vi "Aero_tunnel_monitor_on_OGI.vi"() -> ()   [LabVIEW 2018]
uses:
  Controls/Post_Process.ctl
  <vilib>/Platform/TimedLoop/XDataNode/timing_clust.ctl
  <vilib>/Platform/TimedLoop/XDataNode/nitl_modes.ctl
  <vilib>/Platform/TimedLoop/XDataNode/wakeup.ctl
  ADAM Client/Sub VIs/ADAM Controls/Update_scan_value.ctl
  Globals/Meas_global.vi
  <vilib>/Utility/file.llb/Write Delimited Spreadsheet (DBL).vi
  <vilib>/Platform/TimedLoop/XDataNode/XDataNode.xnode
  <vilib>/Platform/TimedLoop/XDataNode/XDNodeRunTimeDep.lvlib
panel:
  in  "Filename":path
  in  "Duration in Seconds":dbl=30.0
  in  "Log Full Res Balance data":bool
  in  "Use Polynomial for Ratio":bool
  in  "Manual Ratio":dbl=1.0075
  in  "Display Graph?":bool
  in  "Menu Ring":u16(ring) items=["Lift", "Pitch", "Drag", "Side", "Yaw", "Roll"]
  in  "Samples":i32=1000
  out "Waveform Chart":dbl[](graph)
  in  "Output Roll":bool
  out "Roll":string="0.0 Nm"
  in  "Output Yaw":bool
  out "Yaw":string="0.0 Nm"
  in  "Output Pitch":bool
  out "Pitch":string="0.0 Nm"
  in  "Output SF":bool
  out "SF":string="0.0 N"
  in  "Output Drag":bool
  out "Drag":string="0.0 N"
  in  "Output Lift":bool
  out "Lift":string="0.0 N"
  in  "Balance Safety limits":T1(array[cluster])=[{"Max +ve Range"=80, "Max -ve Range"=80, "Axis"="Lift"}, {"Max +ve Range"=80, "Max -ve Range"=80, "Axis"="Pitch"}, {"Max +ve Range"=80, "Max -ve Range"=80, "Axis"="Drag"}, {"Max +ve Range"=80, "Max -ve Range"=80, "Axis"="Side-Force"}, {"Max +ve Range"=99, "Max -ve Range"=99, "Axis"="Yaw"}, {"Max +ve Range"=80, "Max -ve Range"=80, "Axis"="Roll"}] {"Max -ve Range" min=0 max=125; "Max +ve Range" min=0 max=125}
  out "Monitor Speed (Hz)":dbl
  out "Belt slip warning":bool
  out "Road Status":string="???"
  in  "GotoYaw":bool
  in  "NewYawPos":dbl
  out "YAW POSITION":dbl
  out "Required WindSpeedRatio":dbl
  out "ROAD SPEED m/s":dbl
  in  "BL Fan1":i32
  in  "BL Fan2":i32
  in  "Stop drive":bool
  in  "Start Drive":bool
  in  "Synch to Wind":bool
  out "Road Info":string="???"
  in  "stop":bool
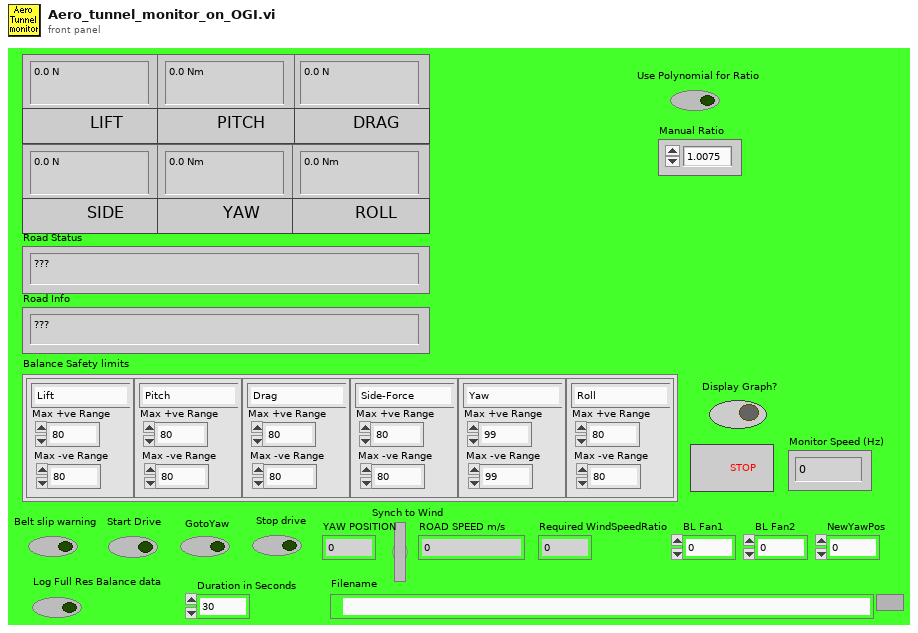
[diagram p1: front panel]
types:
  T1 = cluster{"Max +ve Range":i32, "Max -ve Range":i32, "Axis":string}[]
  T2 = typedef "Post_Process.ctl" = enum16{"Take New Data", "Post Process Raw Data File"}
  T3 = typedef "XDNodeRunTimeDep.lvlib/timing_clust.ctl" = cluster{"Expected End [f-1]":u64, "Actual End [f-1]":u64, "Finished Late? [f-1]":bool, "Expected End [i-1]":u64, "Actual End [i-1]":u64, "Finished Late? [i-1]":bool, "Expected Start [i]":u64, "Actual Start [i]":u64, "Expected Start [f]":u64, "Actual Start [f]":u64, "Source Name":string, "Structure Name":string, "Period":i64, "Deadline":i64, "Offset":i64, "Start":i64, "Priority":i32, "Timeout":i32, "Mode":T4, "Wakeup Reason":T5, "Error":errorcluster, "Source Type":string, "Secondary Source Type":string, "Global End Time":u64, "Global Start Time":u64, "Frame Duration":u64, "Iteration Duration":u64, "Assigned CPU":i32, "I/O Scan Engine Mode":u32}
  T4 = typedef "XDNodeRunTimeDep.lvlib/nitl_modes.ctl" = enum32{"No Change", "Process missed periods, maintain original phase", "Discard missed periods, maintain original phase", "Process missed periods, ignore original phase", "Discard missed periods, ignore original phase"}
  T5 = typedef "XDNodeRunTimeDep.lvlib/wakeup.ctl" = enum32{"Normal", "Aborted", "Asynchronous wakeup", "Timing source error", "Timed loop error", "Timeout"}
  T6 = typedef "Update_scan_value.ctl" = cluster{"Channel Name":string, "New Value":dbl}
  T7 = cluster{"Max +ve Range":i32, "Max -ve Range":i32, "Axis":string}
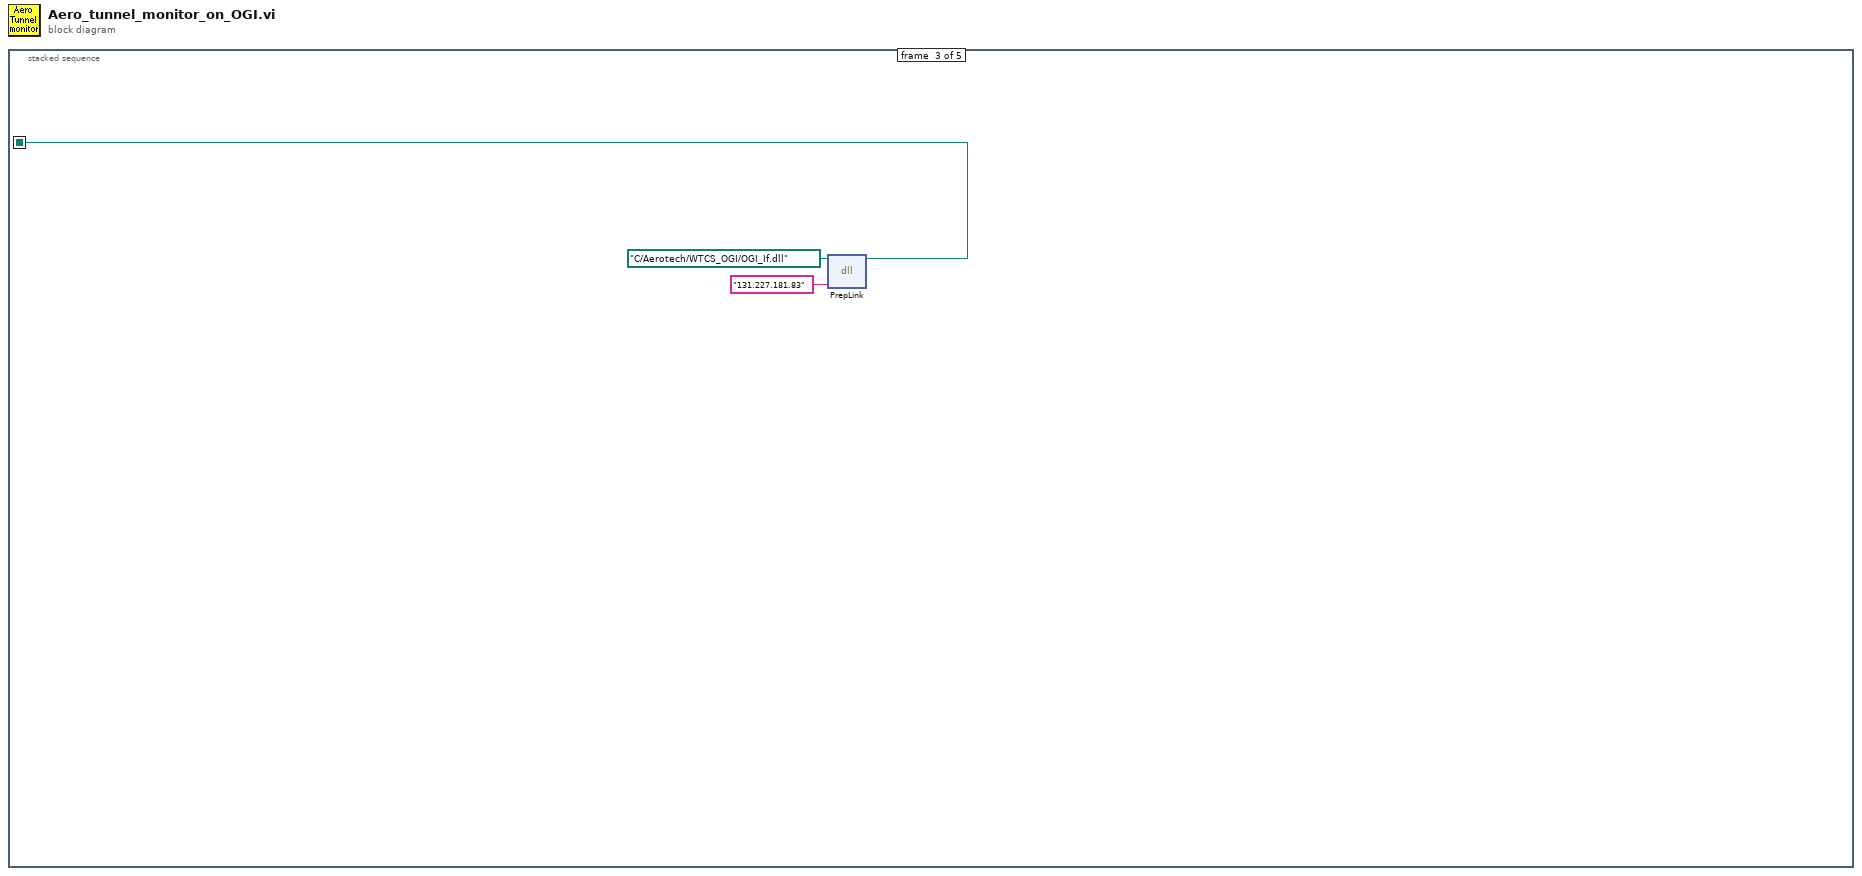
[diagram p0: block diagram]
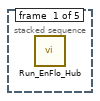
[diagram p2: hidden frame]
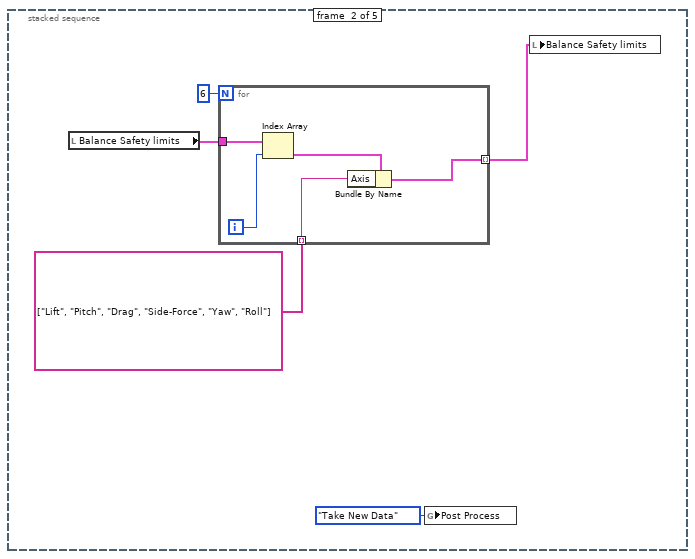
[diagram p3: hidden frame]
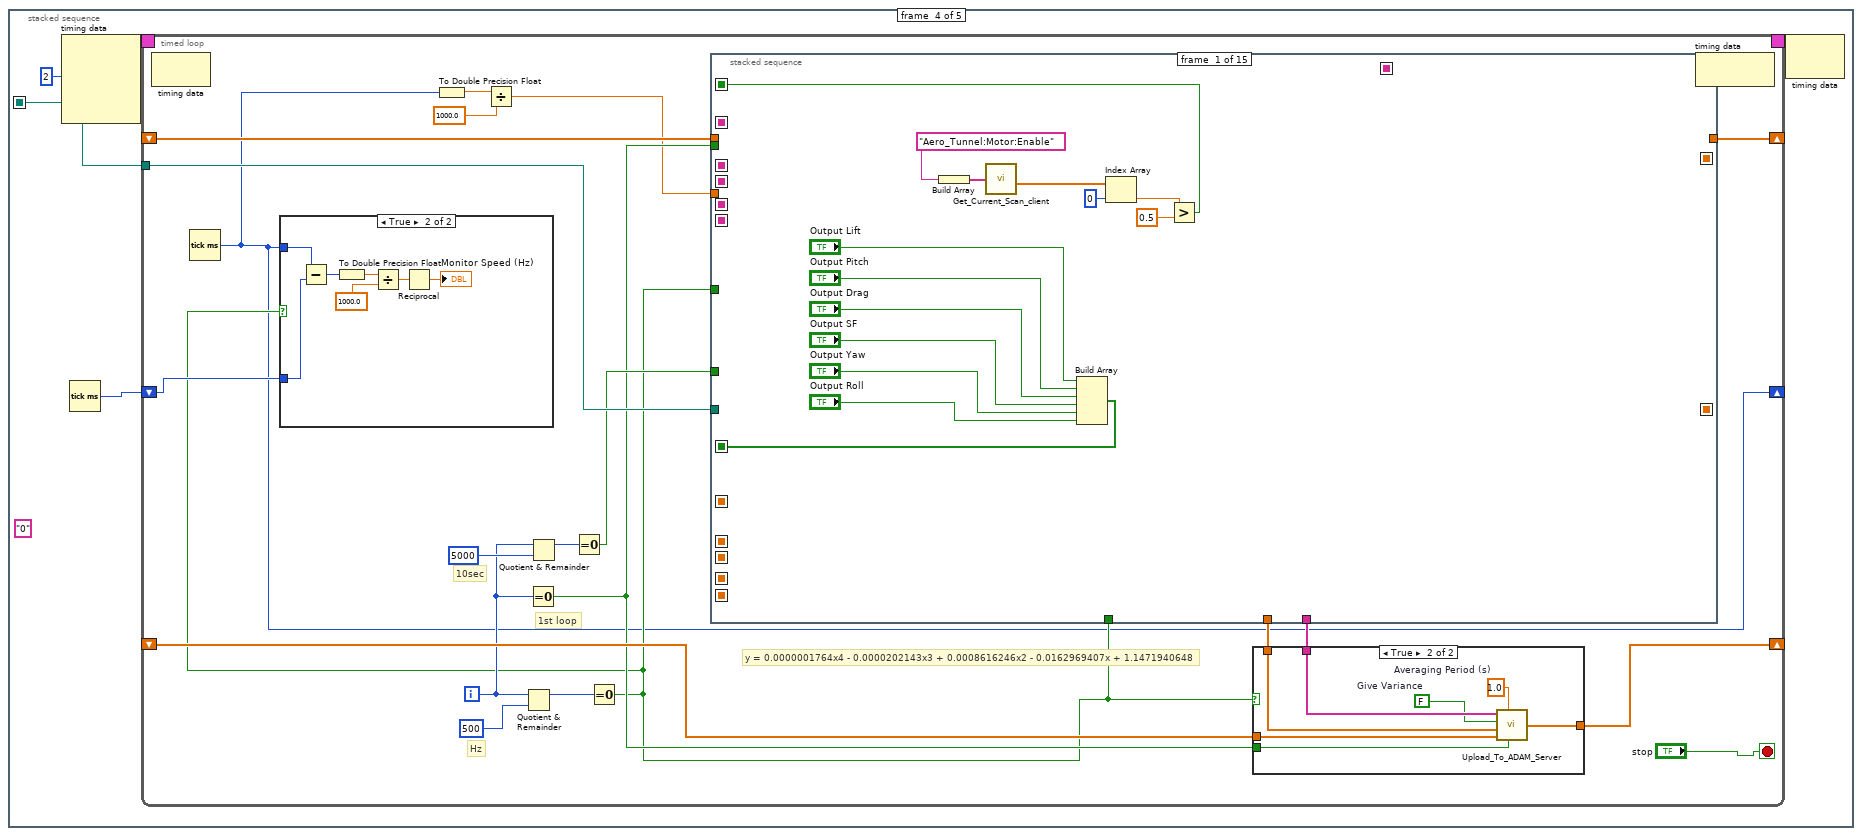
[diagram p4: hidden frame]
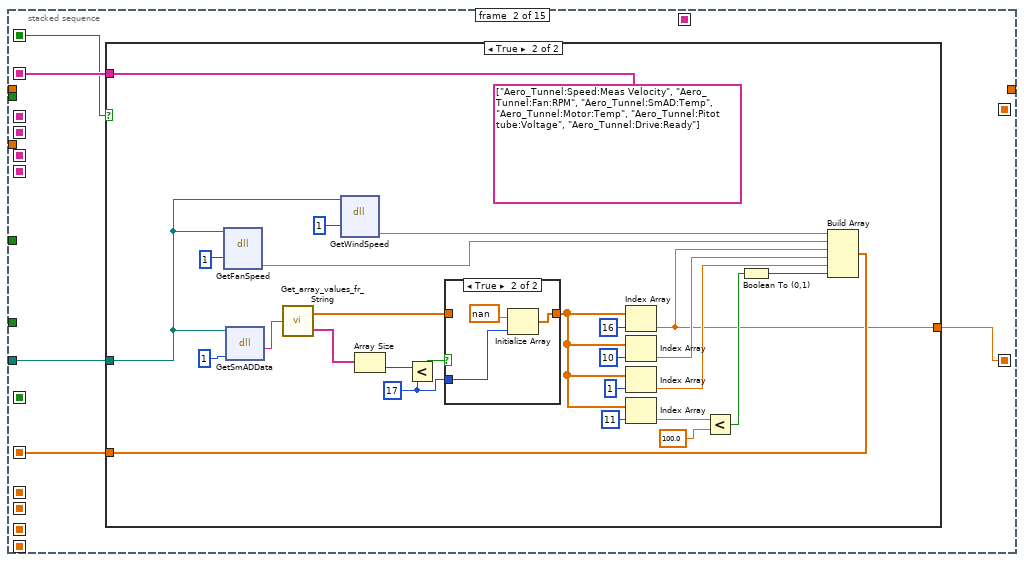
[diagram p7: hidden frame]
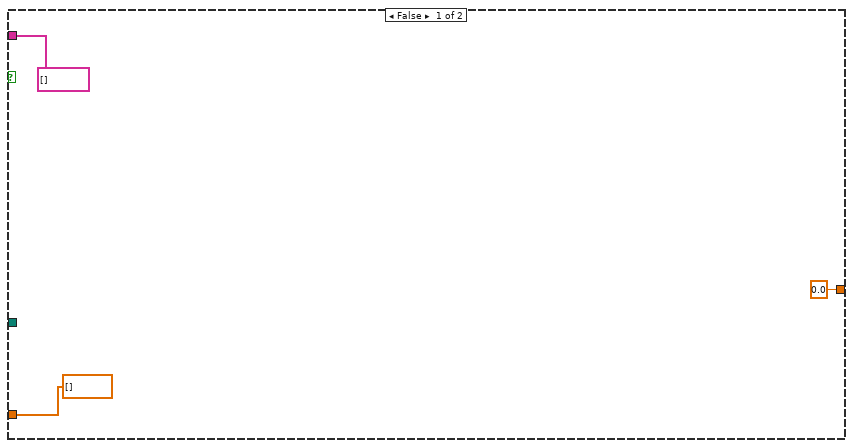
[diagram p8: hidden frame]
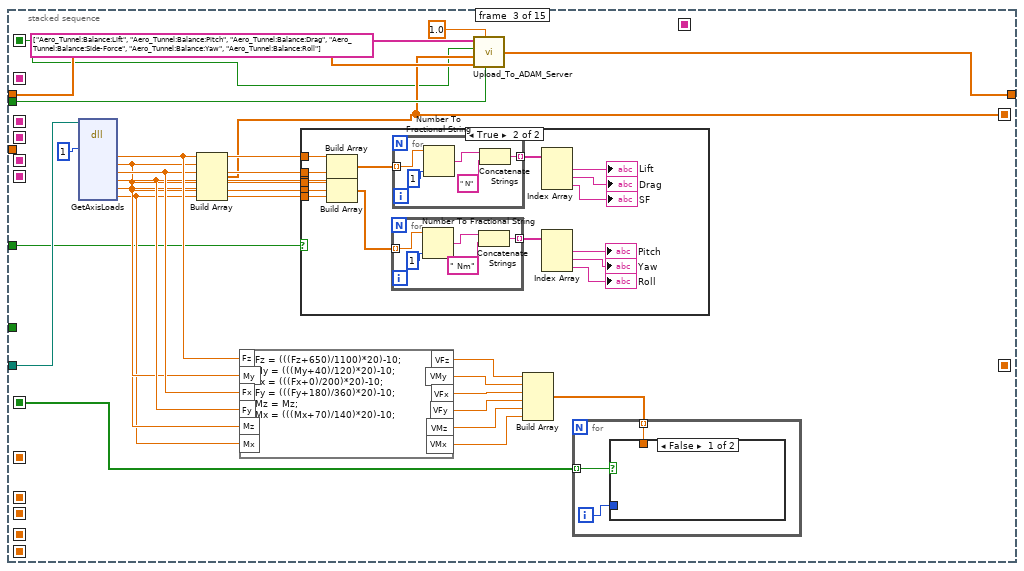
[diagram p10: hidden frame]
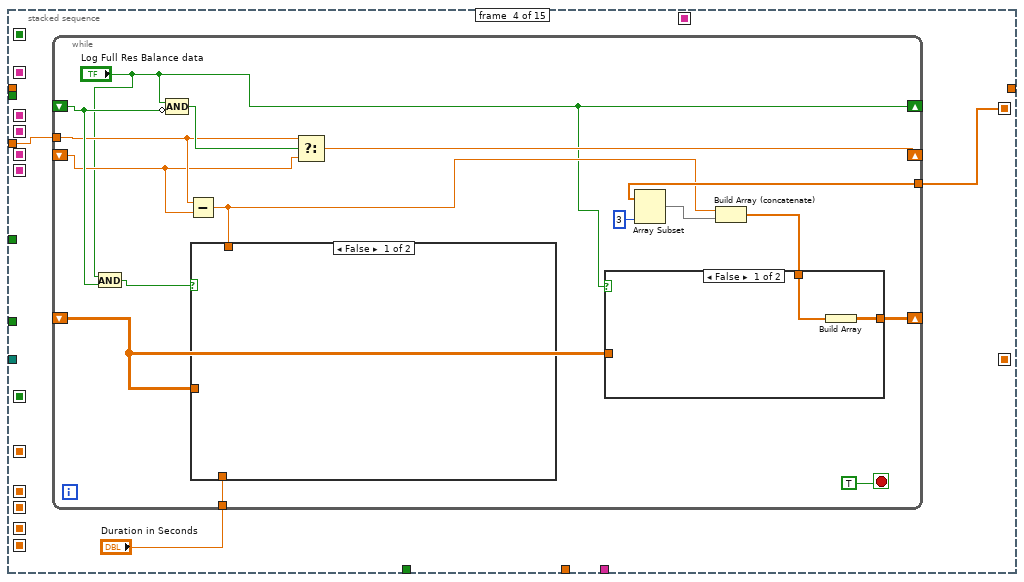
[diagram p13: hidden frame]
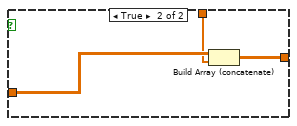
[diagram p14: hidden frame]
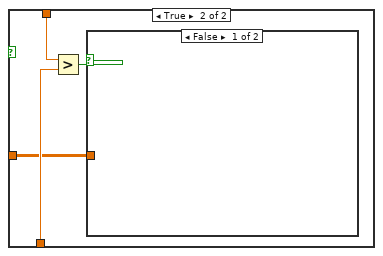
[diagram p15: hidden frame]
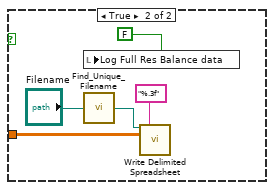
[diagram p16: hidden frame]
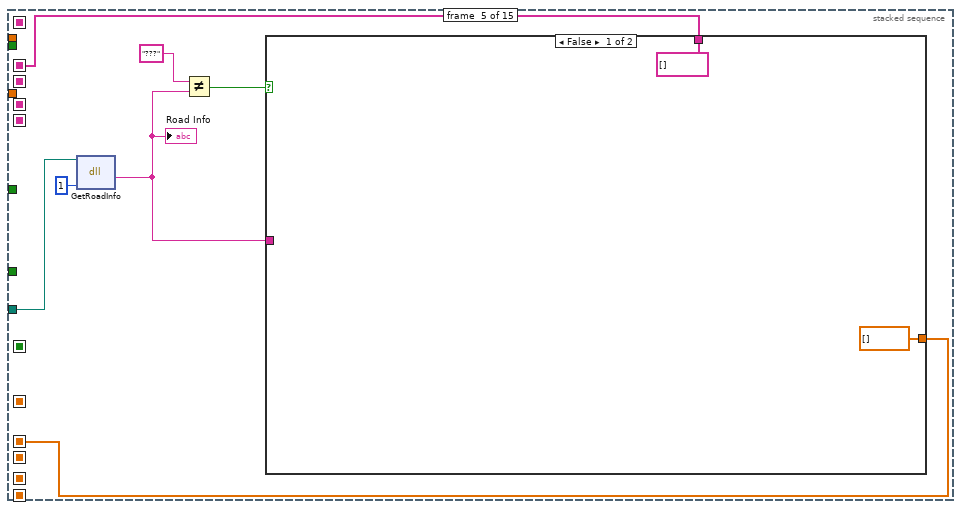
[diagram p17: hidden frame]
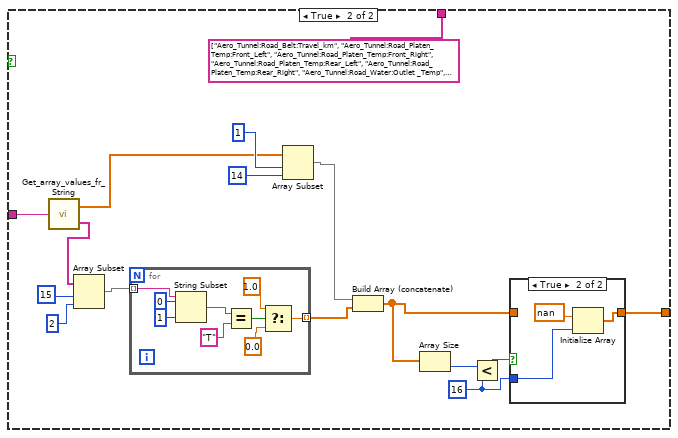
[diagram p18: hidden frame]
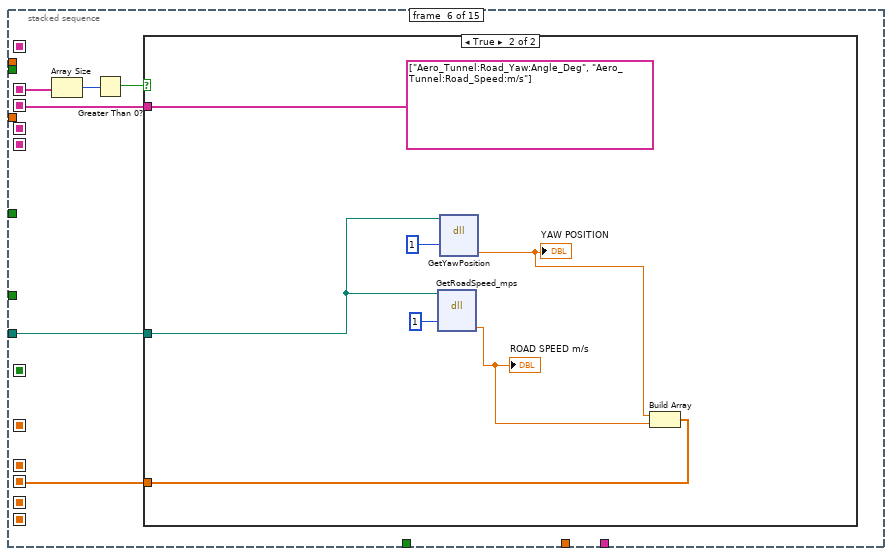
[diagram p20: hidden frame]
diagram:
  n1 = stacked-sequence {
    seq-local: [_ _ w11 _ _] -> [_ _ _ w18 w592]
    frame #0 {
      n2 = call "Run_EnFlo_Hub.vi"() -> ()  [unwired: 7 in, 1 out]
    }
    frame #1 {
      n3 = local read "Balance Safety limits"() -> (w4:T1)
      n4 = for {
        N: 6 -> [_]
        tunnel: w4 -> [w10]
        tunnel: [w7] -> w3 mode=indexing
        tunnel: string[] ["Lift", "Pitch", "Drag", "Side-Force", "Yaw", "Roll"] ("Channel Names") -> [w6] mode=indexing
        i -> [w9]
        n5 = Index Array(array=w10, index=w9) -> (element=w8:T7)
        n6 = Bundle By Name(cluster=w8, "Axis"=w6) -> (w7:T7)
      }
      n7 = global write "Meas_global.vi" "Post Process"(Post_Process."Take New Data" ("Post Process")) -> ()
      n8 = local write "Balance Safety limits"(w3) -> ()
    }
    frame #2 {
      n9 = dll-call lib="C:/Aerotech/Drivers/OGI_IF.dll" fn="PrepLink"(path in=path "C:/Aerotech/WTCS_OGI/OGI_If.dll", "IPAddress"="131.227.181.83") -> (path out=w11:path)  [unwired: 2 in, 3 out]
    }
    frame #3 {
      (unwired) "0" ("Channels")
      n10 = node-c288(i64 2 ("Period")) -> (w16:T3)  [unwired: 3 in]
      n11 = Tick Count (ms)() -> (millisecond timer value=w17:u32)
      n12 = timed-loop {
        shift-right: [w39] -> _
        shift-left: _ -> [w37]
        tunnel: w18 -> [w35]
        shift-right: [w33] -> _
        shift-left: _ -> [w34]
        timing: w16 -> [_]
        timing-out: [_] -> w15
        shift-right: [w22] -> _
        shift-left: w17 -> [w32]
        i -> [w26]
        stop <- "stop" stop-if-true
        # "1st loop"
        # "10sec"
        # "Hz"
        # "y = 0.0000001764x4 - 0.0000202143x3 + 0.0008616246x2 - 0.0162969407x + 1.1471940648"
        n13 = node-c288() -> ()  [unwired: 1 in, 1 out]
        n14 = Tick Count (ms)() -> (millisecond timer value=w22:u32)
        n15 = To Double Precision Float(number=w22) -> (double precision float=w20:dbl)
        n16 = Divide(x=w20, y=1000.0) -> (x/y=w19:dbl)
        n17 = Quotient & Remainder(x=w26, y=500) -> (x-y*floor(x/y)=w29:i32)  [unwired: 1 out]
        n18 = Equal To 0?(x=w26) -> (x = 0?=w25:bool)
        n19 = Quotient & Remainder(x=w26, y=5000) -> (x-y*floor(x/y)=w28:i32)  [unwired: 1 out]
        n20 = Equal To 0?(x=w28) -> (x = 0?=w27:bool)
        n21 = Equal To 0?(x=w29) -> (x = 0?=w24:bool)
        n22 = case shown="True" w24 {
          tunnel: w32 -> [_ w46]
          tunnel: w22 -> [_ w45]
          frame False {
          }
          frame True {
            n23 = Subtract(x=w45, y=w46) -> (x-y=w44:u32)
            n24 = To Double Precision Float(number=w44) -> (double precision float=w40:dbl)
            n25 = Divide(x=w40, y=1000.0) -> (x/y=w42:dbl)
            n26 = Reciprocal(x=w42) -> (1/x=→"Monitor Speed (Hz)":dbl)
          }
        }
        n27 = stacked-sequence {
          seq-local: [_ w74 _ _ _ _ _ _ _ _ _ _ _ _ _] -> [_ _ _ _ _ _ _ _ _ _ _ w398 _ _ _]
          seq-local: [_ w75 _ _ _ _ _ _ _ _ _ _ _ _ _] -> [_ _ _ _ _ _ _ _ _ _ _ w397 _ _ _]
          seq-local: [_ _ _ _ w198 _ _ _ _ _ _ _ _ _ _] -> [_ _ _ _ _ _ _ _ _ _ _ w394 _ _ _]
          seq-local: [_ _ _ _ w199 _ _ _ _ _ _ _ _ _ _] -> [_ _ _ _ _ w235 _ _ _ _ _ w383 _ _ _]
          seq-local: [_ _ _ _ _ w238 _ _ _ _ _ _ _ _ _] -> [_ _ _ _ _ _ _ _ _ _ _ w393 _ _ _]
          seq-local: [_ _ _ _ _ w236 _ _ _ _ _ _ _ _ _] -> [_ _ _ _ _ _ _ _ _ _ _ w392 _ _ _]
          seq-local: [_ _ _ _ _ _ w252 _ _ _ _ _ _ _ _] -> [_ _ _ _ _ _ _ _ _ _ _ w388 _ _ _]
          seq-local: [_ _ _ _ _ _ w251 _ _ _ _ _ _ _ _] -> [_ _ _ _ _ _ _ _ _ _ _ w387 _ _ _]
          seq-local: [w64 _ _ _ _ _ _ _ _ _ _ _ _ _ _] -> [_ _ w124 _ _ _ _ _ _ _ _ _ _ _ _]
          seq-local: [_ _ _ _ _ _ _ w277 _ _ _ _ _ _ _] -> [_ _ _ _ _ _ _ _ _ _ _ w384 _ _ _]
          seq-local: [_ _ _ _ _ _ _ w276 _ _ _ _ _ _ _] -> [_ _ _ _ _ _ _ _ w313 _ _ w385 _ _ _]
          seq-local: [_ _ _ _ _ _ _ _ w309 _ _ _ _ _ _] -> [_ _ _ _ _ _ _ _ _ w343 w362 _ _ _ _]
          seq-local: [_ w72 _ _ _ _ _ _ _ _ _ _ _ _ _] -> [_ _ _ _ _ _ _ _ _ _ w361 _ _ _ _]
          seq-local: [_ _ w110 _ _ _ _ _ _ _ _ _ _ _ _] -> [_ _ _ w162 _ _ _ _ _ _ _ _ _ _ _]
          seq-local: [w57 _ _ _ _ _ _ _ _ _ _ _ _ _ _] -> [_ w71 w109 _ _ _ _ w275 _ _ _ _ _ _ _]
          tunnel: [_ _ _ _ _ _ _ _ _ _ _ w396 _ _ _] -> w38
          tunnel: [_ _ _ _ _ _ _ _ _ _ _ w395 _ _ _] -> w36
          tunnel: w35 -> [_ w73 w131 _ w200 w237 w253 w278 _ _ _ w386 w400 w495 w522]
          tunnel: w24 -> [_ _ _ _ _ _ _ _ _ _ _ _ _ _ _]
          tunnel: w34 -> [_ _ w120 _ _ _ _ _ _ _ _ _ _ _ _]
          tunnel: [_ _ w119 _ _ _ _ _ _ _ _ _ _ _ _] -> w33
          tunnel: w24 -> [_ _ w112 _ _ _ _ _ _ _ _ _ w399 _ w521]
          tunnel: w27 -> [_ _ _ _ _ _ _ _ _ w342 _ _ _ w494 _]
          tunnel: w25 -> [_ _ w111 _ _ _ _ _ _ _ _ _ _ _ _]
          tunnel: w19 -> [_ _ _ w164 _ _ _ _ _ _ _ _ _ _ _]
          frame #0 {
            n28 = Build Array("Aero_Tunnel:Motor:Enable") -> (w62:string[])
            n29 = call "Get_Current_Scan_client.vi"("ADAM Ch Names"=w62) -> ("Numerical Values"=w61:dbl[])  [unwired: 1 in, 2 out]
            n30 = Build Array("Output Lift", "Output Pitch", "Output Drag", "Output SF", "Output Yaw", "Output Roll") -> (w64:bool[])
            n31 = Index Array(array=w61, index=0) -> (element=w59:dbl)
            n32 = Greater?(x=w59, y=0.5) -> (0:w57:bool)
          }
          frame #1 {
            n33 = case shown="True" w71 {
              tunnel: [dbl[] [] w94] -> w75
              tunnel: [string[] [] ("Channel Names") string[] ["Aero_Tunnel:Speed:Meas Velocity", "Aero_Tunnel:Fan:RPM", "Aero_Tunnel:SmAD:Temp", "Aero_Tunnel:Motor:Temp", "Aero_Tunnel:Pitot tube:Voltage", "Aero_Tunnel:Drive:Ready"] ("Channel Names")] -> w74
              tunnel: w73 -> [_ w86]
              tunnel: [0.0 w79] -> w72
              frame False {
              }
              frame True {
                w80 = 17 ("y")
                n34 = dll-call lib="C:/Aerotech/Drivers/OGI_IF.dll" fn="GetFanSpeed"(path in=w86, "Enable"=1) -> ("FanSpeedinRPM"=w88:dbl)  [unwired: 3 in, 4 out]
                n35 = dll-call lib="C:/Aerotech/Drivers/OGI_IF.dll" fn="GetSmADData"(path in=w86, "Enable"=1) -> ("SmAD Data String"=w91:string)  [unwired: 2 in, 3 out]
                n36 = call "Get_array_values_fr_String.vi"("String Value"=w91) -> ("Numeric Array"=w81:dbl[], "String array"=w84:string[])
                n37 = dll-call lib="C:/Aerotech/Drivers/OGI_IF.dll" fn="GetWindSpeed"(path in=w86, "Enable"=1) -> ("Windspeed_M/s"=w87:dbl)  [unwired: 3 in, 4 out]
                n38 = Array Size(array=w84) -> (size(s)=w85:i32)
                n39 = Less?(x=w85, y=w80) -> (x < y?=w83:bool)
                n40 = case shown="True" w83 {
                  tunnel: [w105 w108] -> w82
                  tunnel: w81 -> [w105 _]
                  tunnel: w80 -> [_ w106]
                  frame False {
                  }
                  frame True {
                    n41 = Initialize Array(nan, w106) -> (w108:dbl[])
                  }
                }
                n42 = Index Array(array=w82, index=16) -> (element=w79:dbl)
                n43 = Index Array(array=w82, index=10) -> (element=w102:dbl)
                n44 = Index Array(array=w82, index=1) -> (element=w100:dbl)
                n45 = Index Array(array=w82, index=11) -> (element=w98:dbl)
                n46 = Less?(x=w98, y=100.0) -> (x < y?=w96:bool)
                n47 = Boolean To (0,1)(Boolean=w96) -> (0, 1=w95:i16)
                n48 = Build Array(w87, w88, w79, w102, w100, w95) -> (w94:dbl[])
              }
            }
          }
          frame #2 {
            n49 = dll-call lib="C:/Aerotech/Drivers/OGI_IF.dll" fn="GetAxisLoads"(path in=w131, "Enable"=1) -> ("Lift"=w118:dbl, "Pitch"=w115:dbl, "Drag"=w117:dbl, "side"=w116:dbl, "Yaw"=w114:dbl, "Roll"=w113:dbl)  [unwired: 3 in, 9 out]
            n50 = Build Array(w118, w115, w117, w116, w114, w113) -> (w110:dbl[])
            n51 = formula code="VFz = (((Fz+650)/1100)*20)-10;\nVMy = (((My+40)/120)*20)-10;\nVFx = (((Fx+0)/200)*20)-10;\nVFy = (((Fy+180)/360)*20)-10;\nVMz = Mz;\nVMx = (((Mx+70)/140)*20)-10;"("Fz"=w118, "My"=w115, "Fx"=w117, "Fy"=w116, "Mz"=w114, "Mx"=w113) -> ("VFz"=w130:dbl, "VMy"=w129:dbl, "VFx"=w128:dbl, "VFy"=w127:dbl, "VMz"=w126:dbl, "VMx"=w125:dbl)
            n52 = case shown="True" w112 {
              tunnel: w118 -> [_ w148]
              tunnel: w117 -> [_ w147]
              tunnel: w116 -> [_ w146]
              tunnel: w115 -> [_ w140]
              tunnel: w114 -> [_ w139]
              tunnel: w113 -> [_ w138]
              frame False {
              }
              frame True {
                n53 = Build Array(w148, w147, w146) -> (w145:dbl[])
                n54 = Build Array(w140, w139, w138) -> (w137:dbl[])
                n55 = for {
                  tunnel: w137 -> [w149] mode=indexing
                  tunnel: [w153] -> w136 mode=indexing
                  n56 = Number To Fractional String(number=w149, precision (6)=i16 1) -> (F-format string=w150:string)  [unwired: 2 in]
                  n57 = Concatenate Strings(w150, " Nm" ("string")) -> (w153:string)
                }
                n58 = for {
                  tunnel: w145 -> [w154] mode=indexing
                  tunnel: [w158] -> w144 mode=indexing
                  n59 = Number To Fractional String(number=w154, precision (6)=i16 1) -> (F-format string=w155:string)  [unwired: 2 in]
                  n60 = Concatenate Strings(w155, " N" ("string")) -> (w158:string)
                }
                n61 = Index Array(array=w144) -> (element #1=→"Lift":string, element #2=→"Drag":string, element #3=→"SF":string)  [unwired: 3 in]
                n62 = Index Array(array=w136) -> (element #1=→"Pitch":string, element #2=→"Yaw":string, element #3=→"Roll":string)  [unwired: 3 in]
              }
            }
            n63 = call "Upload_To_ADAM_Server.vi"("First Loop"=w111, "Averaging Period (s)"=1.0, "Shift In"=w120, "Channel Values"=w110, "Give Variance"=w109, "Channel Names"=string[] ["Aero_Tunnel:Balance:Lift", "Aero_Tunnel:Balance:Pitch", "Aero_Tunnel:Balance:Drag", "Aero_Tunnel:Balance:Side-Force", "Aero_Tunnel:Balance:Yaw", "Aero_Tunnel:Balance:Roll"]) -> ("Shift Out"=w119:dbl[])
            n64 = Build Array(w130, w129, w128, w127, w126, w125) -> (w123:dbl[])
            n65 = for {
              tunnel: w124 -> [w161] mode=indexing
              tunnel: w123 -> [w160] mode=indexing
              i -> [w159]
              n66 = case shown="False" w161 {
                tunnel: w160 -> [_ _]
                tunnel: w159 -> [_ _]
                frame False {
                }
                frame True {
                }
              }
            }
          }
          frame #3 {
            n67 = while {
              shift-right: ["Log Full Res Balance data"] -> _
              shift-left: _ -> [w178]
              shift-right: [w179] -> _
              shift-left: _ -> [w172]
              tunnel: w164 -> [w173]
              tunnel: "Duration in Seconds" -> [w176]
              tunnel: w162 -> [w174]
              shift-right: [w170] -> _
              shift-left: _ -> [w165]
              stop <- TRUE stop-if-true
              n68 = And(x="Log Full Res Balance data", y=w178) -> (x .and. y?=w177:bool)
              n69 = Compound Arithmetic op=AND("Log Full Res Balance data", invert w178) -> (w180:bool)
              n70 = Subtract(x=w173, y=w172) -> (x-y=w171:dbl)
              n71 = case shown="False" w177 {
                tunnel: w176 -> [_ w189]
                tunnel: w171 -> [_ w187]
                tunnel: w165 -> [_ w186]
                frame False {
                }
                frame True {
                  n72 = Greater?(x=w187, y=w189) -> (0:w188:bool)
                  n73 = case shown="False" w188 {
                    tunnel: w186 -> [_ w193]
                    frame False {
                    }
                    frame True {
                      n74 = local write "Log Full Res Balance data"(FALSE) -> ()
                      n75 = call "Find_Unique_Filename.vi"("Path In"="Filename") -> ("Unique Path Out"=w191:path)  [unwired: 2 in]
                      n76 = call-poly <vilib>:"Write Delimited Spreadsheet.vi"("file path (dialog if empty)"=w191, "format (%.3f)"="%.3f", "2D data"=w193) -> ()  [unwired: 11 in, 2 out]
                    }
                  }
                }
              }
              n77 = Select(t=w173, s=w180, f=w172) -> (s? t:f=w179:dbl)
              n78 = Array Subset(array=w174, length=3) -> (w168:dbl[])  [unwired: 1 in]
              n79 = Build Array (concatenate)(w171, w168) -> (w167:dbl[])
              n80 = case shown="False" "Log Full Res Balance data" {
                tunnel: [w181 w185] -> w170
                tunnel: w165 -> [_ w184]
                tunnel: w167 -> [w182 w183]
                frame False {
                  n81 = Build Array(w182) -> (w181:dbl[][])
                }
                frame True {
                  n82 = Build Array (concatenate)(w184, w183) -> (w185:dbl[][])
                }
              }
            }
          }
          frame #4 {
            n83 = dll-call lib="C:/Aerotech/Drivers/OGI_IF.dll" fn="GetRoadInfo"(path in=w200, "Enable"=1) -> ("Road Info"=w196:string)  [unwired: 3 in, 2 out]
            "Road Info" <- w196
            n84 = Not Equal?(x="???", y=w196) -> (x != y?=w195:bool)
            n85 = case shown="False" w195 {
              tunnel: [string[] [] ("Channel Names") string[] ["Aero_Tunnel:Road_Belt:Travel_km", "Aero_Tunnel:Road_Platen_Temp:Front_Left", "Aero_Tunnel:Road_Platen_Temp:Front_Right", "Aero_Tunnel:Road_Platen_Temp:Rear_Left", "Aero_Tunnel:Road_Platen_Temp:Rear_Right", "Aero_Tunnel:Road_Water:Outlet _Temp", "Aero_Tunnel:Road_Water:Inlet _Temp", "Aero_Tunnel:Road_Suction:Front", "Aero_Tunnel:Road_Suction:Middle", "Aero_Tunnel:Road_Suction:Rear", "Aero_Tunnel:Road_BL_Suction:Primary", "Aero_Tunnel:Road_BL_Suction:Secondary", "Aero_Tunnel:Road_LoadCell:Left", "Aero_Tunnel:Road_LoadCell:Right", "Aero_Tunnel:Road_Water_High:Temp_Alarm", "Aero_Tunnel:Road_Platen_High:Temp_Alarm"] ("Channel Names")] -> w199
              tunnel: [dbl[] [] w205] -> w198
              tunnel: w196 -> [_ w204]
              frame False {
              }
              frame True {
                w208 = 16 ("y")
                n86 = call "Get_array_values_fr_String.vi"("String Value"=w204) -> ("Numeric Array"=w207:dbl[], "String array"=w211:string[])
                n87 = Array Subset(array=w211, index=15, length=2) -> (w215:string[])
                n88 = for {
                  tunnel: w215 -> [w230] mode=indexing
                  tunnel: [w224] -> w214 mode=indexing
                  n89 = String Subset(string=w230, offset (0)=0, length (rest)=1 ("length (rest)")) -> (substring=w229:string)
                  n90 = Equal?(x=w229, y="T") -> (x = y?=w227:bool)
                  n91 = Select(t=1.0, s=w227, f=0.0) -> (s? t:f=w224:dbl)
                }
                n92 = Array Subset(array=w207, index=1, length=14) -> (w213:dbl[])
                n93 = Build Array (concatenate)(w213, w214) -> (w206:dbl[])
                n94 = Array Size(array=w206) -> (size(s)=w210:i32)
                n95 = Less?(x=w210, y=w208) -> (x < y?=w209:bool)
                n96 = case shown="True" w209 {
                  tunnel: [w220 w223] -> w205
                  tunnel: w206 -> [w220 _]
                  tunnel: w208 -> [_ w221]
                  frame False {
                  }
                  frame True {
                    n97 = Initialize Array(nan, w221) -> (w223:dbl[])
                  }
                }
              }
            }
          }
          frame #5 {
            n98 = Array Size(array=w235) -> (size(s)=w234:i32)
            n99 = Greater Than 0?(x=w234) -> (x > 0?=w233:bool)
            n100 = case shown="True" w233 {
              tunnel: [string[] [] ("Channel Names") string[] ["Aero_Tunnel:Road_Yaw:Angle_Deg", "Aero_Tunnel:Road_Speed:m/s"] ("Channel Names")] -> w238
              tunnel: w237 -> [_ w244]
              tunnel: [dbl[] [] w241] -> w236
              frame False {
              }
              frame True {
                n101 = dll-call lib="C:/Aerotech/Drivers/OGI_IF.dll" fn="GetRoadSpeed_mps"(path in=w244, "Enable"=1) -> ("RoadSpeed_mps"=w242:dbl)  [unwired: 3 in, 4 out]
                "ROAD SPEED m/s" <- w242
                n102 = dll-call lib="C:/Aerotech/Drivers/OGI_IF.dll" fn="GetYawPosition"(path in=w244, "Enable"=1) -> ("Yaw Position"=w243:dbl)  [unwired: 3 in, 4 out]
                "YAW POSITION" <- w243
                n103 = Build Array(w243, w242) -> (w241:dbl[])
              }
            }
          }
          frame #6 {
            n104 = dll-call lib="C:/Aerotech/Drivers/OGI_IF.dll" fn="GetRoadStatus"(path in=w253, "Enable"=1) -> ("Road Status"=w250:string)  [unwired: 3 in, 2 out]
            "Road Status" <- w250
            n105 = Not Equal?(x="???", y=w250) -> (x != y?=w248:bool)
            n106 = case shown="False" w248 {
              tunnel: [string[] [] ("Channel Names") string[] ["Aero_Tunnel:Road_E-Stop:Active", "Aero_Tunnel:Road_Main_Drives:Started", "Aero_Tunnel:Road_Belt_Slip:Warning", "Aero_Tunnel:Road_Belt_Absent:or_Broken", "Aero_Tunnel:Road_Suction:Established", "Aero_Tunnel:Road_Load_Error:Left", "Aero_Tunnel:Road_Load_Error:Right", "Aero_Tunnel:Road_Water_Alarm:Active", "Aero_Tunnel:Road_Platen_Alarm:Active"] ("Channel Names")] -> w252
              tunnel: [dbl[] [] w264] -> w251
              tunnel: w250 -> [_ w257]
              frame False {
              }
              frame True {
                n107 = call "Get_array_values_fr_String.vi"("String Value"=w257) -> ("String array"=w260:string[])  [unwired: 1 out]
                n108 = Array Subset(array=w260, index=1) -> (w258:string[])  [unwired: 1 in]
                n109 = for {
                  tunnel: [w267] -> w264 mode=indexing
                  tunnel: w258 -> [w266] mode=indexing
                  n110 = String Subset(string=w266, offset (0)=0, length (rest)=1 ("length (rest)")) -> (substring=w272:string)
                  n111 = Equal?(x=w272, y="T") -> (x = y?=w270:bool)
                  n112 = Select(t=1.0, s=w270, f=0.0) -> (s? t:f=w267:dbl)
                }
                n113 = Index Array(array=w264, index=2) -> (element=w262:dbl)
                n114 = Greater Than 0?(x=w262) -> (x > 0?=→"Belt slip warning":bool)
              }
            }
          }
          frame #7 {
            n115 = case shown="True" w275 {
              tunnel: w278 -> [_ w291]
              tunnel: [string[] [] ("Channel Names") string[] ["Aero_Tunnel:Balance_Range:Lift", "Aero_Tunnel:Balance_Range:Pitch", "Aero_Tunnel:Balance_Range:Drag", "Aero_Tunnel:Balance_Range:Side-Force", "Aero_Tunnel:Balance_Range:Yaw", "Aero_Tunnel:Balance_Range:Roll"] ("Channel Names")] -> w277
              tunnel: [dbl[] [] w282] -> w276
              frame False {
              }
              frame True {
                n116 = dll-call lib="C:/Aerotech/Drivers/OGI_IF.dll" fn="GetAxisPercs"(path in=w291, "Enable"=1) -> ("Lift"=w289:dbl, "Pitch"=w288:dbl, "Drag"=w287:dbl, "side"=w286:dbl, "Yaw"=w285:dbl, "Roll"=w284:dbl)  [unwired: 3 in, 9 out]
                n117 = Build Array(w289, w288, w287, w286, w285, w284) -> (w282:dbl[])
                n118 = case shown="False" "Display Graph?" {
                  selector: "Display Graph?" -> [w292 w293]
                  tunnel: w282 -> [_ w297]
                  frame False {
                    n119 = property on="Waveform Chart" class="WFChart (strict)"("Visible"=w292) -> ()  [unwired: 2 in, 2 out]
                    n120 = property on="Samples" class="DigNum (strict)"("Visible"=w292) -> ()  [unwired: 2 in, 2 out]
                    n121 = property on="Menu Ring" class="Ring (strict)"("Visible"=w292) -> ()  [unwired: 2 in, 2 out]
                  }
                  frame True {
                    n122 = while {
                      shift-right: [w299] -> _
                      shift-left: _ -> [w301]
                      tunnel: w297 -> [w300]
                      tunnel: [w299] -> w296
                      stop <- TRUE stop-if-true
                      n123 = for {
                        tunnel: w301 -> [w304]
                        tunnel: w300 -> [w302] mode=indexing
                        tunnel: [w307] -> w299 mode=indexing
                        i -> [w305]
                        n124 = Index Array(array=w304, index (row)=w305) -> (element=w303:dbl[])  [unwired: 1 in]
                        n125 = Build Array (concatenate)(w302, w303) -> (w308:dbl[])
                        n126 = Array Subset(array=w308, length="Samples") -> (w307:dbl[])  [unwired: 1 in]
                      }
                    }
                    n127 = Index Array(array=w296, index (row)="Menu Ring") -> (element=→"Waveform Chart":dbl[])  [unwired: 1 in]
                    n128 = property on="Waveform Chart" class="WFChart (strict)"("Visible"=w293) -> ()  [unwired: 2 in, 2 out]
                    n129 = property on="Samples" class="DigNum (strict)"("Visible"=w293) -> ()  [unwired: 2 in, 2 out]
                    n130 = property on="Menu Ring" class="Ring (strict)"("Visible"=w293) -> ()  [unwired: 2 in, 2 out]
                  }
                }
              }
            }
          }
          frame #8 {
            n131 = for {
              tunnel: "Balance Safety limits" -> [w329] mode=indexing
              tunnel: w313 -> [w332] mode=indexing
              shift-right: [w326] -> w310
              shift-left: "" -> [w327]
              n132 = To Long Integer(number=w332) -> (32bit integer=w328:i32)
              n133 = Unbundle By Name(w329) -> ("Max +ve Range"=w334:i32, "Max -ve Range"=w333:i32)
              n134 = Negate(x=w333) -> (-x=w331:i32)
              n135 = In Range and Coerce(upper limit=w334, x=w328, lower limit=w331) -> (In Range?=w330:bool)  [unwired: 1 out]
              n136 = case shown="False" w330 {
                tunnel: w329 -> [w340 _]
                tunnel: w328 -> [w338 _]
                tunnel: w327 -> [w336 w341]
                tunnel: [w335 w341] -> w326
                frame False {
                  n137 = Unbundle By Name(w340) -> ("Axis"=w339:string)
                  n138 = Format Into String(format string="The %s is at %d%% of its range.\n", initial string=w336, w339, w338) -> (resulting string=w335:string)  [unwired: 1 in, 1 out]
                }
                frame True {
                }
              }
            }
            n139 = Empty String/Path?(string/path=w310) -> (empty?=w311:bool)
            n140 = case shown="False" w311 {
              tunnel: w310 -> [w317 w325]
              tunnel: [w315 w325] -> w309
              frame False {
                n141 = Build Array("Aero_Tunnel:Fan:Watchdog") -> (w324:string[])
                n142 = call "Get_Current_Scan_client.vi"("ADAM Ch Names"=w324) -> ("Numerical Values"=w322:dbl[])  [unwired: 1 in, 2 out]
                n143 = Index Array(array=w322, index=0) -> (element=w320:dbl)
                n144 = Greater?(x=w320, y=0.5) -> (0:w318:bool)
                n145 = Select(t=w317, s=w318, f="") -> (s? t:f=w315:string)
              }
              frame True {
              }
            }
          }
          frame #9 {
            n146 = while {
              tunnel: w343 -> [w347]
              tunnel: w342 -> [w344]
              stop <- TRUE stop-if-true
              n147 = Empty String/Path?(string/path=w347) -> (empty?=w349:bool)
              n148 = Not(x=w349) -> (.not. x?=w345:bool)
              n149 = Compound Arithmetic op=AND(w345, w344) -> (w348:bool)
              n150 = case shown="False" w348 {
                tunnel: w347 -> [_ w354]
                frame False {
                }
                frame True {
                  w353 = string[] ["Aero_Tunnel:Fan:Watchdog", "Aero_Tunnel:Road:Watchdog", "Aero_Tunnel:Speed:Dem Velocity"] ("Channel Names")
                  n151 = Format Into String(format string="The Aero Tunnel balance has gone outside of its limits.\n%s\nThe Aero_Tunnel:Fan:Watchdog has therefore been disabled. ", w354) -> (resulting string=w355:string)  [unwired: 2 in, 1 out]
                  n152 = Bundle By Name(cluster=errorcluster {"status"=TRUE, "code"=0, "source"=""} ("error in (no error)"), "source"=w355) -> (w357:errorcluster)
                  n153 = Array Size(array=w353) -> (size(s)=w352:i32)
                  n154 = call "EnFlo_Error_Handler.vi"("error in (no error)"=w357, "Error Type"="Aero Tunnel Balance Range Trip", "Dialog Box (T)"=FALSE) -> ()  [unwired: 3 out]
                  n155 = Initialize Array(0.0, w352) -> (w350:dbl[])
                  n156 = call "ASYNC_Adam_client.vi"("Values"=w350, "Channel Names"=w353) -> ()  [unwired: 1 in, 2 out]
                }
              }
            }
          }
          frame #10 {
            n157 = while {
              tunnel: w362 -> [_]
              shift-right: [w367] -> _
              shift-left: _ -> [w366]
              tunnel: w361 -> [w364]
              stop <- TRUE stop-if-true
              n158 = Greater?(x=w364, y=35.0) -> (0:w367:bool)
              n159 = Number To Fractional String(number=w364, precision (6)=i16 2) -> (F-format string=w363:string)  [unwired: 2 in]
              n160 = Compound Arithmetic op=AND(invert w366, w367) -> (w370:bool)
              n161 = case shown="True" w370 {
                tunnel: w363 -> [_ w375]
                frame False {
                }
                frame True {
                  w374 = string[] ["Aero_Tunnel:Fan:Watchdog", "Aero_Tunnel:Road:Watchdog", "Aero_Tunnel:Speed:Dem Velocity"] ("Channel Names")
                  n162 = Format Into String(format string="The Aero Tunnel temperature has gone above it's limits and is:\n%s\nThe Aero_Tunnel:Fan:Watchdog has therefore been disabled. ", w375) -> (resulting string=w376:string)  [unwired: 2 in, 1 out]
                  n163 = Bundle By Name(cluster=errorcluster {"status"=TRUE, "code"=0, "source"=""} ("error in (no error)"), "source"=w376) -> (w378:errorcluster)
                  n164 = Array Size(array=w374) -> (size(s)=w373:i32)
                  n165 = call "EnFlo_Error_Handler.vi"("error in (no error)"=w378, "Error Type"="Aero Tunnel Temperature Trip", "Dialog Box (T)"=FALSE) -> ()  [unwired: 3 out]
                  n166 = Initialize Array(0.0, w373) -> (w371:dbl[])
                  n167 = call "ASYNC_Adam_client.vi"("Values"=w371, "Channel Names"=w374) -> ()  [unwired: 1 in, 2 out]
                }
              }
            }
          }
          frame #11 {
            n168 = Build Array (concatenate)(w397, w394, w392, w387, w385) -> (w396:dbl[])
            n169 = Boolean To (0,1)(Boolean="GotoYaw") -> (0, 1=w391:i16)
            n170 = Build Array (concatenate)(w398, w383, w393, w388, w384) -> (w395:string[])
            n171 = To Long Integer(number=w391) -> (32bit integer=w382:i32)
            n172 = dll-call lib="C:/Aerotech/Drivers/OGI_IF.dll" fn="GotoYawPosition"(path in=w386, "Enable"=w382, "NewYawPos"="NewYawPos") -> ()  [unwired: 3 in, 4 out]
          }
          frame #12 {
            n173 = case shown="True" w399 {
              tunnel: w400 -> [_ w401]
              frame False {
              }
              frame True {
                # "Tweak"
                # "Speed"
                # "Tweak"
                # "Speed"
                n174 = stacked-sequence {
                  seq-local: [_ w415 _ _ _ _] -> [_ _ _ w460 _ _]
                  seq-local: [_ w406 _ _ _ _] -> [_ _ _ w456 _ _]
                  seq-local: [_ w413 _ _ _ _] -> [_ _ _ _ w476 _]
                  seq-local: [_ w409 _ _ _ _] -> [_ _ _ _ _ w485]
                  seq-local: [_ w407 _ _ _ _] -> [_ _ _ _ _ _]
                  seq-local: [_ w405 _ _ _ _] -> [_ _ _ _ _ _]
                  seq-local: [string[] ["Aero_Tunnel:Speed:Dem Velocity", "Froude:NPL:Atmos_Press", "Aero_Tunnel:Motor:Enable", "Aero_Tunnel:Speed:Calib Tweak", "Aero_Tunnel:Upper:Temp", "Aero_Tunnel:Lower:Temp", "Aero_Tunnel:Fan:Watchdog"] ("appended array") _ _ _ _ _] -> [_ w404 _ _ _ _]
                  seq-local: [_ w403 _ _ _ _] -> [_ _ w439 _ _ _]
                  tunnel: w401 -> [_ w417 _ w459 w475 w486]
                  frame #0 {
                  }
                  frame #1 {
                    n175 = call "Get_Current_Scan_client.vi"("ADAM Ch Names"=w404) -> ("Numerical Values"=w403:dbl[])  [unwired: 1 in, 2 out]
                    n176 = Index Array(array=w403, index=0) -> (element=w415:dbl)
                    n177 = Index Array(array=w403, index=3) -> (element=w407:dbl)
                    n178 = Index Array(array=w403, index=1) -> (element=w413:dbl)
                    n179 = while {
                      tunnel: w417 -> [w425]
                      tunnel: w415 -> [w424]
                      shift-right: [w424] -> _
                      shift-left: _ -> [w423]
                      shift-right: [w420] -> _
                      shift-left: _ -> [w421]
                      tunnel: w407 -> [w420]
                      tunnel: [w419] -> w406
                      tunnel: [w418] -> w405
                      stop <- TRUE stop-if-true
                      n180 = Not Equal?(x=w424, y=w423) -> (x != y?=w419:bool)
                      n181 = Not Equal?(x=w420, y=w421) -> (x != y?=w418:bool)
                      n182 = case shown="False" w419 {
                        tunnel: w425 -> [_ w426]
                        tunnel: w424 -> [_ w427]
                        frame False {
                        }
                        frame True {
                          n183 = Greater?(x=w427, y=0.2) -> (0:w428:bool)
                          n184 = Boolean To (0,1)(Boolean=w428) -> (0, 1=w431:i16)
                          n185 = dll-call lib="C:/Aerotech/Drivers/OGI_IF.dll" fn="SetFanSystemState"(path in=w426, "Enable"=1, "Fan ONOFF"=w431) -> ()  [unwired: 3 in, 4 out]
                        }
                      }
                    }
                    n186 = Index Array(array=w403, index=2) -> (element=w411:dbl)
                    n187 = Greater?(x=w411, y=0.5) -> (0:w409:bool)
                  }
                  frame #2 {
                    # "allowed temp."
                    n188 = Index Array(array=w439, index=6) -> (element=w437:dbl)
                    n189 = Array Subset(array=w439, index=4, length=3) -> (w441:dbl[])
                    n190 = Array Max & Min(array=w441) -> (max value=w432:dbl)  [unwired: 3 out]
                    n191 = Greater?(x=w437, y=0.5) -> (0:w434:bool)
                    n192 = Greater?(x=w432, y=35.0) -> (0:w435:bool)
                    n193 = And(x=w435, y=w434) -> (x .and. y?=w433:bool)
                    n194 = case shown="False" w433 {
                      tunnel: w432 -> [_ w446]
                      frame False {
                      }
                      frame True {
                        n195 = Format Into String(format string="Aero Tunnel temp is %.1f. The Aero_Tunnel:Fan:Watchdog has therefore been disabled. ", w446) -> (resulting string=w444:string)  [unwired: 2 in, 1 out]
                        n196 = Bundle By Name(cluster=errorcluster {"status"=TRUE, "code"=0, "source"=""} ("error in (no error)"), "source"=w444) -> (w447:errorcluster)
                        n197 = call "EnFlo_Error_Handler.vi"("error in (no error)"=w447, "Error Type"="Aero Tunnel over temp", "Dialog Box (T)"=FALSE) -> ()  [unwired: 3 out]
                        n198 = call "ASYNC_Adam_client.vi"("Values"=dbl[] [0.0, 0.0], "Channel Names"=string[] ["Aero_Tunnel:Fan:Watchdog", "Aero_Tunnel:Road:Watchdog"]) -> ()  [unwired: 1 in, 2 out]
                      }
                    }
                  }
                  frame #3 {
                    n199 = feedback-in #1("Manual Ratio") -> ()
                    n200 = feedback #1() -> (w458:dbl)  [unwired: 1 in]
                    n201 = Not Equal?(x="Manual Ratio", y=w458) -> (x != y?=w454:bool)
                    n202 = Or(x=w454, y=w456) -> (x .or. y?=w455:bool)
                    n203 = case shown="False" w455 {
                      tunnel: w460 -> [_ w468]
                      tunnel: w459 -> [_ w474]
                      tunnel: "Manual Ratio" -> [_ w462]
                      tunnel: "Use Polynomial for Ratio" -> [_ w464]
                      frame False {
                      }
                      frame True {
                        (unwired) dbl[] [0.7807, 0.0283, -0.0013, 2e-05] ("Calib constants")
                        # "no fillets no rolling road no suction"
                        # "rolling road full suction fillets"
                        n204 = call "Polynomial_convert.vi"("Calib constants"=dbl[] [1.1471940648, -0.0162969407, 0.0008616246, -2.02143e-05, 1.764e-07], "Voltage"=w468) -> ("Eng Values"=w463:dbl)  [unwired: 4 in]
                        n205 = Select(t=w463, s=w464, f=w462) -> (s? t:f=w461:dbl)
                        n206 = Equal To 0?(x=w468) -> (x = 0?=w469:bool)
                        n207 = In Range and Coerce(upper limit=1.12, x=w461, lower limit=0.88) -> (coerced(x)=w466:dbl)  [unwired: 1 out]
                        n208 = Select(t=0.88, s=w469, f=w466) -> (s? t:f=w465:dbl)
                        "Required WindSpeedRatio" <- w465
                        n209 = dll-call lib="C:/Aerotech/Drivers/OGI_IF.dll" fn="SetWindSpeedRatio"(path in=w474, "Enable"=1 ("t"), "Required WindSpeedRatio"=w465) -> ()  [unwired: 4 in, 3 out]
                      }
                    }
                  }
                  frame #4 {
                    n210 = while {
                      shift-right: [w478] -> _
                      shift-left: _ -> [w481]
                      tunnel: w476 -> [w478]
                      tunnel: w475 -> [w479]
                      stop <- TRUE stop-if-true
                      n211 = Equal?(x=w478, y=w481) -> (x = y?=w480:bool)
                      n212 = case shown="True" w480 {
                        tunnel: w479 -> [_ w484]
                        tunnel: w478 -> [_ w482]
                        frame False {
                        }
                        frame True {
                          n213 = dll-call lib="C:/Aerotech/Drivers/OGI_IF.dll" fn="SetNewbaroPr_mB"(path in=w484, "Enable"=1, "NewPressure"=w482) -> ()  [unwired: 3 in, 4 out]
                        }
                      }
                    }
                  }
                  frame #5 {
                    n214 = while {
                      shift-right: [w489] -> _
                      shift-left: _ -> [w488]
                      tunnel: w485 -> [w489]
                      tunnel: w486 -> [w491]
                      stop <- TRUE stop-if-true
                      n215 = Compound Arithmetic op=AND(w489, invert w488) -> (w487:bool)
                      n216 = case shown="True" w487 {
                        tunnel: w491 -> [_ w493]
                        frame False {
                        }
                        frame True {
                          n217 = dll-call lib="C:/Aerotech/Drivers/OGI_IF.dll" fn="SetPitotZero"(path in=w493, "Enable"=1) -> ()  [unwired: 2 in, 4 out]
                        }
                      }
                    }
                  }
                }
              }
            }
          }
          frame #13 {
            n218 = while {
              tunnel: w495 -> [w502]
              shift-right: [w500] -> _
              shift-left: _ -> [w499]
              tunnel: w494 -> [w498]
              shift-right: [w496] -> _
              shift-left: _ -> [w497]
              stop <- TRUE stop-if-true
              # "Do every 10 seconds"
              n219 = case shown="False" w498 {
                tunnel: w502 -> [_ _]
                tunnel: [w504 w518] -> w500
                tunnel: w499 -> [w504 w517]
                tunnel: w497 -> [w503 w509]
                tunnel: [w503 w507] -> w496
                frame False {
                  (unwired) FALSE
                }
                frame True {
                  # "Do every 10 minutes"
                  # "flip flop every 10 cycles"
                  n220 = Increment(x=w509) -> (x+1=w506:i32)
                  n221 = Greater?(x=w506, y=60) -> (0:w505:bool)
                  n222 = case shown="False" w505 {
                    tunnel: [w519 0] -> w507
                    tunnel: w506 -> [w519 _]
                    frame False {
                    }
                    frame True {
                    }
                  }
                  n223 = Select(t=1.0, s=w517, f=0.0) -> (s? t:f=w511:dbl)
                  n224 = Bundle By Name(cluster=T6 {"Channel Name"="Aero_Tunnel:Server:Pulse", "New Value"=0.0} ("Update Scan Value Cluster"), "New Value"=w511) -> (w513:T6)
                  n225 = Not(x=w517) -> (.not. x?=w518:bool)
                  n226 = Build Array(w513) -> (w512:T6[])
                  n227 = call "Update_Current_Value_client.vi"("Don't Bother with check?"=TRUE, "Update array in"=w512) -> ()
                }
              }
            }
          }
          frame #14 {
            n228 = while {
              shift-right: [w533] -> _
              shift-left: _ -> [w535]
              tunnel: w521 -> [w534]
              tunnel: w522 -> [w531]
              shift-right: [w529] -> _
              shift-left: _ -> [w530]
              shift-right: [w527] -> _
              shift-left: _ -> [w528]
              shift-right: [w524] -> _
              shift-left: _ -> [w526]
              shift-right: [w523] -> _
              shift-left: _ -> [w525]
              stop <- TRUE stop-if-true
              n229 = stacked-sequence {
                tunnel: w535 -> [w541 _ _ _]
                tunnel: w534 -> [w539 w557 w567 w579]
                tunnel: ["Synch to Wind" _ _ _] -> w533
                tunnel: w531 -> [w536 w555 w565 w581]
                tunnel: w530 -> [_ w554 _ _]
                tunnel: [_ "Start Drive" _ _] -> w529
                tunnel: w528 -> [_ _ w564 _]
                tunnel: [_ _ "Stop drive" _] -> w527
                tunnel: w526 -> [_ _ _ w578]
                tunnel: w525 -> [_ _ _ w575]
                tunnel: [_ _ _ "BL Fan1"] -> w524
                tunnel: [_ _ _ "BL Fan2"] -> w523
                frame #0 {
                  n230 = Not Equal?(x="Synch to Wind", y=w541) -> (x != y?=w540:bool)
                  n231 = Or(x=w540, y=w539) -> (x .or. y?=w537:bool)
                  n232 = case shown="False" w537 {
                    tunnel: "Synch to Wind" -> [_ w550]
                    tunnel: w536 -> [w542 w549]
                    frame False {
                      n233 = Build Array("Aero_Tunnel:Road:Dem_Velocity") -> (w546:string[])
                      n234 = call "Get_Current_Scan_client.vi"("ADAM Ch Names"=w546) -> ("Numerical Values"=w545:dbl[])  [unwired: 1 in, 2 out]
                      n235 = Index Array(array=w545) -> (element=w544:dbl)  [unwired: 1 in]
                      n236 = dll-call lib="C:/Aerotech/Drivers/OGI_IF.dll" fn="SetRoadSpeed_mps"(path in=w542, "Enable"=1, "Required_mps"=w544) -> ()  [unwired: 3 in, 4 out]
                    }
                    frame True {
                      n237 = Boolean To (0,1)(Boolean=w550) -> (0, 1=w551:i16)
                      n238 = To Long Integer(number=w551) -> (32bit integer=w548:i32)
                      n239 = dll-call lib="C:/Aerotech/Drivers/OGI_IF.dll" fn="RoadSyncToWind"(path in=w549, "Enable"=1, "SynchState"=w548) -> ()  [unwired: 3 in, 4 out]
                    }
                  }
                }
                frame #1 {
                  n240 = Not Equal?(x="Start Drive", y=w554) -> (x != y?=w558:bool)
                  n241 = Or(x=w558, y=w557) -> (x .or. y?=w556:bool)
                  n242 = case shown="True" w556 {
                    tunnel: "Start Drive" -> [_ w562]
                    tunnel: w555 -> [_ w560]
                    frame False {
                    }
                    frame True {
                      n243 = Boolean To (0,1)(Boolean=w562) -> (0, 1=w561:i16)
                      n244 = To Long Integer(number=w561) -> (32bit integer=w559:i32)
                      n245 = dll-call lib="C:/Aerotech/Drivers/OGI_IF.dll" fn="StartRoadDrive"(path in=w560, "Enable"=w559) -> ()  [unwired: 2 in, 4 out]
                    }
                  }
                }
                frame #2 {
                  n246 = Not Equal?(x="Stop drive", y=w564) -> (x != y?=w568:bool)
                  n247 = Or(x=w568, y=w567) -> (x .or. y?=w566:bool)
                  n248 = case shown="True" w566 {
                    tunnel: "Stop drive" -> [_ w572]
                    tunnel: w565 -> [_ w570]
                    frame False {
                    }
                    frame True {
                      n249 = Boolean To (0,1)(Boolean=w572) -> (0, 1=w571:i16)
                      n250 = To Long Integer(number=w571) -> (32bit integer=w569:i32)
                      n251 = dll-call lib="C:/Aerotech/Drivers/OGI_IF.dll" fn="RoadStop"(path in=w570, "Enable"=w569) -> ()  [unwired: 2 in, 4 out]
                    }
                  }
                }
                frame #3 {
                  n252 = Not Equal?(x=w575, y="BL Fan2") -> (x != y?=w576:bool)
                  n253 = Not Equal?(x="BL Fan1", y=w578) -> (x != y?=w577:bool)
                  n254 = Compound Arithmetic op=OR(w577, w576, w579) -> (w580:bool)
                  n255 = case shown="True" w580 {
                    tunnel: w581 -> [_ w583]
                    tunnel: "BL Fan1" -> [_ w585]
                    tunnel: "BL Fan2" -> [_ w584]
                    frame False {
                    }
                    frame True {
                      w582 = 1 ("BL Fan (1 or 2)")
                      n256 = dll-call lib="C:/Aerotech/Drivers/OGI_IF.dll" fn="SetBoundaryPerc"(path in=w583, "enable"=w582, "BL Fan (1 or 2)"=1, "New Percentage"=w585) -> ()  [unwired: 4 in, 4 out]
                      n257 = dll-call lib="C:/Aerotech/Drivers/OGI_IF.dll" fn="SetBoundaryPerc"(path in=w583, "enable"=w582, "BL Fan (1 or 2)"=2, "New Percentage"=w584) -> ()  [unwired: 4 in, 4 out]
                    }
                  }
                }
              }
            }
          }
        }
        n258 = case shown="True" w24 {
          tunnel: [w49 w56] -> w39
          tunnel: w38 -> [_ w55]
          tunnel: w37 -> [w49 w54]
          tunnel: w36 -> [_ w53]
          tunnel: w25 -> [_ w50]
          frame False {
          }
          frame True {
            w51 = FALSE  # Give Variance
            w52 = 1.0  # Averaging Period (s)
            n259 = call "Upload_To_ADAM_Server.vi"("First Loop"=w50, "Averaging Period (s)"=w52, "Shift In"=w54, "Channel Values"=w55, "Give Variance"=w51, "Channel Names"=w53) -> ("Shift Out"=w56:dbl[])
          }
        }
        n260 = node-c288() -> ()  [unwired: 1 in, 1 out]
      }
      n261 = node-c288(w15) -> ()  [unwired: 1 out]
    }
    frame #4 {
      n262 = dll-call lib="C:/Aerotech/Drivers/OGI_IF.dll" fn="CloseLink"(path in=w592) -> ()  [unwired: 2 in, 3 out]
    }
  }
